vi "Read Limit Test Results.vi"(8 "error in (no error)":errorcluster, 11 "VISA resource name":refnum<visa-resource-name>) -> (0 "error out":errorcluster, 1 "?":T1(array[cluster]) {"lower limit" format="%.3e"; "upper limit" format="%.3e"; "test results" items=["no test", "test failed", "test passed"]; "stimulus value" format="%^.2e"}, 3 "VISA resource name out":refnum<visa-resource-name>)   [LabVIEW 2018, in "Agilent 87XX Series.lvlib"]
doc: "This VI for the HP8753 Network Analyzer is used to read back the results of limit tests. \n\n Units are standard units of Hz, dB, seconds, ohms, etc.\n\n This VI can be used to read the exact stimulus values rather than using the \"Read Stimulus Values\" VI which will sometimes do approximations."
uses:
  Agilent 87XX Series.lvlib
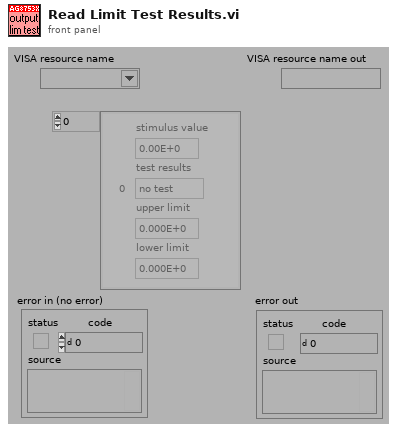
[diagram p1: front panel]
types:
  T1 = cluster{"stimulus value":dbl, "test results":i32, "upper limit":dbl, "lower limit":dbl}[]
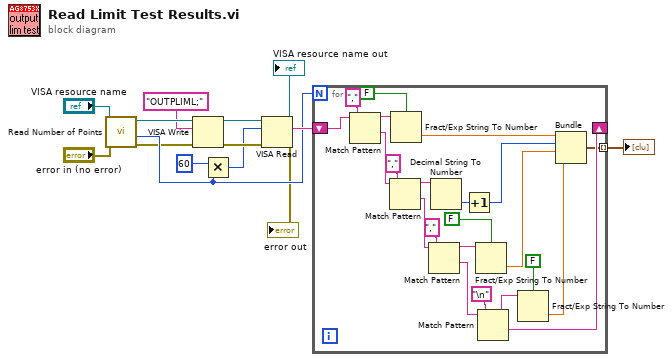
[diagram p0: block diagram]
diagram:
  n1 = call "Read Number of Points.vi"("error in (no error)"="error in (no error)", "VISA resource name"="VISA resource name") -> ("error out"=w6:errorcluster, "num points"=w7:i32, "VISA resource name out"=w14:refnum<visa-resource-name>)  [unwired: 7 in]
  n2 = VISA Write(VISA resource name=w14, write buffer="OUTPLIML;", error in (no error)=w6) -> (VISA resource name out=w2:refnum<visa-resource-name>, error out=w5:errorcluster)  [unwired: 1 out]
  n3 = Multiply(x=u32 60, y=w7) -> (x*y=w1:u32)
  n4 = VISA Read(VISA resource name=w2, byte count=w1, error in (no error)=w5) -> (VISA resource name out=→"VISA resource name out":refnum<visa-resource-name>, read buffer=w12:string, error out=→"error out":errorcluster)  [unwired: 1 out]
  n5 = for {
    N: w7 -> [_]
    shift-right: [w26] -> _
    shift-left: w12 -> [w36]
    tunnel: [w18] -> w11 mode=indexing
    n6 = Match Pattern(string=w36, regular expression=",") -> (before substring=w29:string, after substring=w31:string)  [unwired: 1 in, 2 out]
    n7 = Match Pattern(string=w31, regular expression=",") -> (before substring=w28:string, after substring=w30:string)  [unwired: 1 in, 2 out]
    n8 = Fract/Exp String To Number(use system decimal point (T)=FALSE, string=w29) -> (number=w23:dbl)  [unwired: 2 in, 1 out]
    n9 = Match Pattern(string=w30, regular expression=",") -> (before substring=w25:string, after substring=w27:string)  [unwired: 1 in, 2 out]
    n10 = Decimal String To Number(string=w28) -> (number=w22:i32)  [unwired: 2 in, 1 out]
    n11 = Increment(x=w22) -> (x+1=w21:i32)
    n12 = Fract/Exp String To Number(use system decimal point (T)=FALSE, string=w25) -> (number=w20:dbl)  [unwired: 2 in, 1 out]
    n13 = Match Pattern(string=w27, regular expression="\n") -> (before substring=w24:string, after substring=w26:string)  [unwired: 1 in, 2 out]
    n14 = Fract/Exp String To Number(use system decimal point (T)=FALSE, string=w24) -> (number=w19:dbl)  [unwired: 2 in, 1 out]
    n15 = Bundle(w23, w21, w20, w19) -> (w18:cluster{dbl, i32, dbl, dbl})  [unwired: 1 in]
  }
  "?" <- w11
